vi "SRS 925 Set Channel.vi"(8 "error in":errorcluster, 10 "Cahnnel":i32, 11 "VISA resource name":refnum<visa-resource-name>) -> (0 "error out":errorcluster, 3 "VISA resource name out":refnum<visa-resource-name>)   [LabVIEW 2023]
uses:
  GPIB/VISA  Send Receive.vi
  Simple VISA Reader/Simple VISA Reader Driver.lvclass
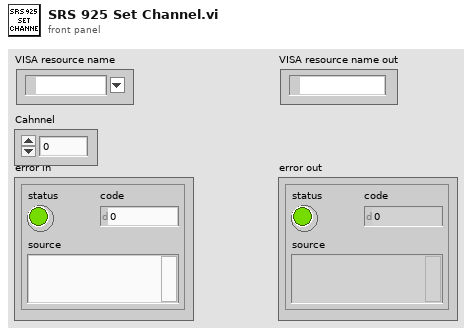
[diagram p1: front panel]
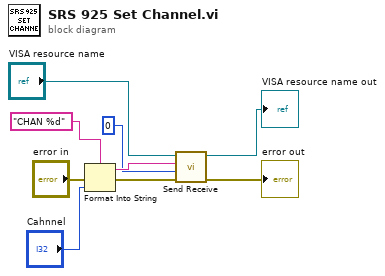
[diagram p0: block diagram]
diagram:
  n1 = Format Into String(format string="CHAN %d", error in="error in", "Cahnnel") -> (resulting string=w2:string, error out=w3:errorcluster)  [unwired: 1 in]
  n2 = call-poly "Send Receive.vi"("error in (no error)"=w3, "Receive count"=0, "data string in"=w2, "VISA Resource Name"="VISA resource name") -> ("error out"=→"error out":errorcluster, "VISA Resource Name Out"=→"VISA resource name out":refnum<visa-resource-name>)  [unwired: 5 in, 1 out]
